vi "Update.vi"(8 "error in (no error)":errorcluster, 10 "Message in":refnum<class "UpdateMessage.lvclass">, 11 "AOTF in":refnum<class "AOTF.lvclass">) -> (0 "error out":errorcluster, 3 "AOTF out":refnum<class "AOTF.lvclass">)   [LabVIEW 2012, in "AOTF.lvclass"]
doc: "The update method processes the command 'update'. \n\nThe command 'update' is used for receiving new values to be set to the private data of the class. This could be seen as a public set method for setting new parameters to the private class data."
uses:
  AOTF.lvclass
  <vilib>/Distrio/Murmex/UpdateMessage/UpdateMessage.lvclass
  AOTF.lvclass/AOTF.ctl
  Controls/laser line ring.ctl
  <vilib>/Distrio/Murmex/Murmex/Murmex.lvclass
panel:
  # "This method is called when the UPDATE\ntrigger is sent. \n\nOverride this method when your component needs to\nrespond to this trigger. \n\nCall parent for proper implementation"
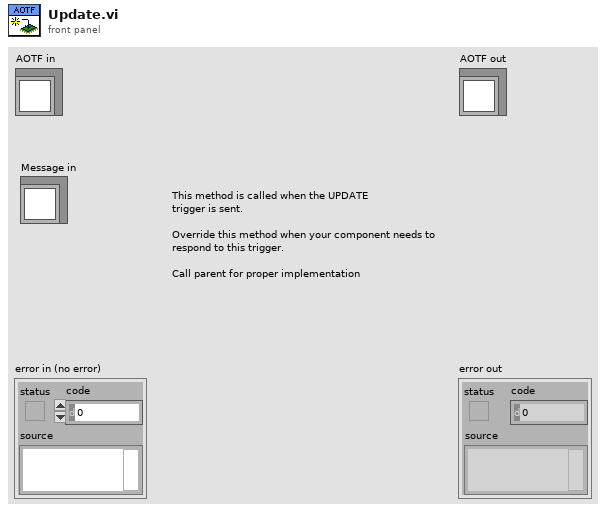
[diagram p1: front panel]
types:
  T1 = typedef "AOTF.lvclass/laser line ring.ctl" = u8
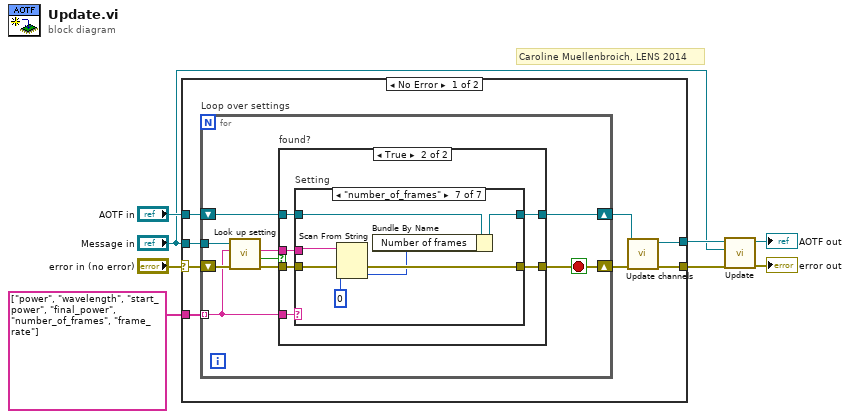
[diagram p0: block diagram]
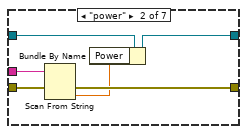
[diagram p4: hidden frame]
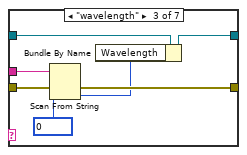
[diagram p5: hidden frame]
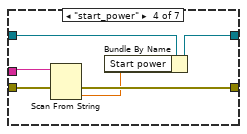
[diagram p6: hidden frame]
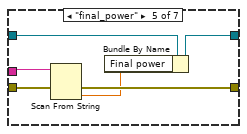
[diagram p7: hidden frame]
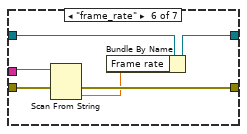
[diagram p8: hidden frame]
diagram:
  # "Caroline Muellenbroich, LENS 2014"
  n1 = case shown="No Error" "error in (no error)" {
    selector: "error in (no error)" -> [w16 w74]
    tunnel: string[] ["power", "wavelength", "start_power", "final_power", "number_of_frames", "frame_rate"] ("key chains") -> [w15 _]
    tunnel: "Message in" -> [w14 _]
    tunnel: "AOTF in" -> [w13 w75]
    tunnel: [w10 w74] -> w3
    tunnel: [w12 w75] -> w2
    frame No Error {
      n2 = for "Loop over settings" {
        shift-right: [w19] -> w9
        shift-left: w16 -> [w25]
        tunnel: w15 -> [w20] mode=indexing
        tunnel: w14 -> [w24]
        shift-right: [w17] -> w11
        shift-left: w13 -> [w18]
        stop <- w19 stop-if-true
        n3 = call <vilib>:"Look up setting.vi"("error in (no error)"=w25, "tag name"=w20, "UpdateMessage in"=w24) -> ("error out"=w21:errorcluster, "found?"=w23:bool, "value"=w22:string)  [unwired: 5 in, 1 out]
        n4 = case "found?" shown="True" w23 {
          tunnel: w22 -> [_ w32]
          tunnel: w21 -> [w27 w31]
          tunnel: w20 -> [_ w33]
          tunnel: [w27 w30] -> w19
          tunnel: w18 -> [w26 w29]
          tunnel: [w26 w28] -> w17
          frame False {
          }
          frame True {
            n5 = case "Setting" shown="\"number_of_frames\"" w33 {
              tunnel: w32 -> [_ w39 w47 w52 w58 w64 w71]
              tunnel: w31 -> [w35 w38 w48 w54 w60 w66 w73]
              tunnel: [w35 w37 w44 w53 w59 w65 w72] -> w30
              tunnel: w29 -> [w34 w41 w46 w51 w57 w63 w70]
              tunnel: [w34 w40 w45 w50 w56 w62 w69] -> w28
              frame Default {
              }
              frame "power" {
                n6 = Scan From String(input string=w39, error in=w38) -> (error out=w37:errorcluster, output 1=w36:dbl)  [unwired: 3 in, 2 out]
                n7 = Bundle By Name(cluster=w41, "Power"=w36) -> (w40:refnum<class "AOTF.lvclass">)
              }
              frame "wavelength" {
                w42 = T1 0 items=["405nm"=1, "445nm"=5, "491nm"=2, "515nm"=3, "561nm"=4] ("Settings cluster.Wavelength")
                n8 = Scan From String(input string=w47, error in=w48, default 1=w42) -> (error out=w44:errorcluster, output 1=w43:T1)  [unwired: 2 in, 2 out]
                n9 = Bundle By Name(cluster=w46, "Wavelength"=w43) -> (w45:refnum<class "AOTF.lvclass">)
              }
              frame "start_power" {
                n10 = Scan From String(input string=w52, error in=w54) -> (error out=w53:errorcluster, output 1=w49:dbl)  [unwired: 3 in, 2 out]
                n11 = Bundle By Name(cluster=w51, "Start power"=w49) -> (w50:refnum<class "AOTF.lvclass">)
              }
              frame "final_power" {
                n12 = Scan From String(input string=w58, error in=w60) -> (error out=w59:errorcluster, output 1=w55:dbl)  [unwired: 3 in, 2 out]
                n13 = Bundle By Name(cluster=w57, "Final power"=w55) -> (w56:refnum<class "AOTF.lvclass">)
              }
              frame "frame_rate" {
                n14 = Scan From String(input string=w64, error in=w66) -> (error out=w65:errorcluster, output 1=w61:dbl)  [unwired: 3 in, 2 out]
                n15 = Bundle By Name(cluster=w63, "Frame rate"=w61) -> (w62:refnum<class "AOTF.lvclass">)
              }
              frame "number_of_frames" {
                n16 = Scan From String(input string=w71, error in=w73, default 1=0 ("Settings cluster.Number of frames")) -> (error out=w72:errorcluster, output 1=w68:i32)  [unwired: 2 in, 2 out]
                n17 = Bundle By Name(cluster=w70, "Number of frames"=w68) -> (w69:refnum<class "AOTF.lvclass">)
              }
            }
          }
        }
      }
      n18 = call-dynamic "Update channels.vi"("error in (no error)"=w9, "AOTF in"=w11) -> ("error out"=w10:errorcluster, "AOTF out"=w12:refnum<class "AOTF.lvclass">)  [unwired: 8 in]
    }
    frame Error {
    }
  }
  n19 = call-parent "Update.vi"("error in (no error)"=w3, "Message in"="Message in", "Murmex in"=w2) -> ("error out"=→"error out":errorcluster, "Murmex out"=→"AOTF out":refnum<class "AOTF.lvclass">)  [unwired: 7 in]
